vi "Epoch Library -- VI Tree.vi"() -> ()   [LabVIEW 2018]
uses:
  <vilib>/LabVIEW Open Source Project/Epoch Date & Time/Epochs -- enum.ctl
  <vilib>/LabVIEW Open Source Project/Epoch Date & Time/formatter.iso8601/ISO8601 Date Formats.ctl
  <vilib>/LabVIEW Open Source Project/Epoch Date & Time/Timestamp Compare Units -- enum.ctl
  <vilib>/LabVIEW Open Source Project/Epoch Date & Time/formatter.iso8601/DateTime.ISO8601.lvclass
  C:/Program Files (x86)/National Instruments/LabVIEW 2018/vi.lib/LabVIEW Open Source Project/Epoch Date & Time/formatter/DateTimeFormatter.lvclass
  <vilib>/LabVIEW Open Source Project/Epoch Date & Time/formatter.rfc5322/DateTime.RFC5322.lvclass
  <vilib>/LabVIEW Open Source Project/Epoch Date & Time/epoch/Epoch.lvclass
  <vilib>/LabVIEW Open Source Project/Epoch Date & Time/epoch.UTC/Epoch.UTC.lvclass
  <vilib>/LabVIEW Open Source Project/Epoch Date & Time/epoch.GPS/Epoch.GPS.lvclass
  C:/Program Files (x86)/National Instruments/LabVIEW 2018/vi.lib/LabVIEW Open Source Project/Epoch Date & Time/epoch/Epoch.lvclass
  <vilib>/LabVIEW Open Source Project/Epoch Date & Time/epoch.UNIX/Epoch.UNIX.lvclass
  <vilib>/LabVIEW Open Source Project/Epoch Date & Time/formatter.iso8601/DateTime.ISO8601.lvclass/DateTime.ISO8601.ctl
  <vilib>/LabVIEW Open Source Project/Epoch Date & Time/isLeapYear (timestamp).vi
  <vilib>/LabVIEW Open Source Project/Epoch Date & Time/isLeapYear (integer).vi
  <vilib>/LabVIEW Open Source Project/Epoch Date & Time/formatter/DateTimeFormatter.lvclass
panel:
  out "Valid RFC5332 Internet Date":bool
  out "UNIX Conversion":bool
  out "UNIX Time (s)":i64
  out "GPS Time (s)":i64
  out "GPS Conversion":bool
  out "RFC5322 Email DateTime String":string
  out "Timestamp":timestamp
  out "ISO Strings":string[](array[string])
  out "timestamps":timestamp[](array[timestamp]) format="%<%.3X %x>T"
  out "Fractional Seconds":dbl[](array[numeric])
  out "Epoch Times (s)":i64[](array[numeric])
  out "Epochs":T1[](array[typedef])=[enum."Local", enum."UTC", enum."Unix", enum."GPS"]
  out "is 2021 a Leap Year?":bool
  out "ISO Week-Day Notation":bool
  out "ISO DateTime Notation":bool
  out "ISO8601 UTC DateTime String":string
  out "Valid RFC3339 Dates":bool
  out "Valid ISO Dates":bool
  out "is 2020 a Leap Year?":bool
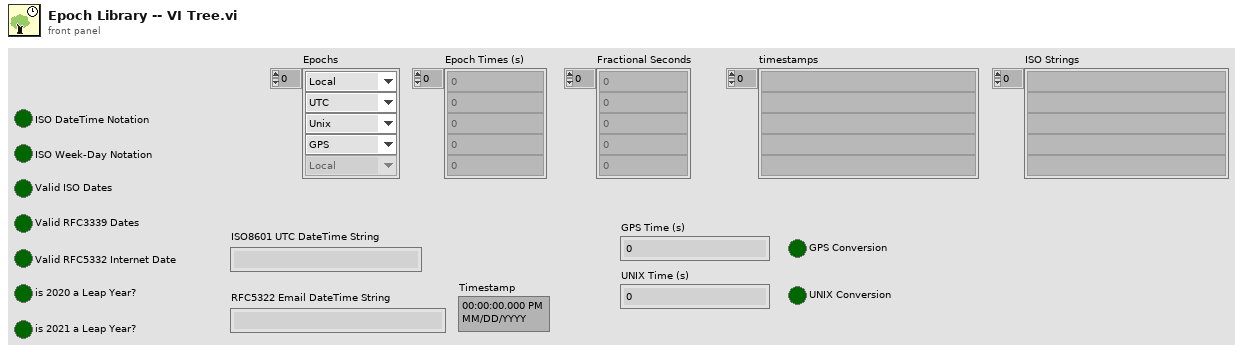
[diagram p1: front panel]
types:
  T1 = typedef "Epochs -- enum.ctl" = enum16{"Local", "UTC", "Unix", "GPS"}
  T2 = typedef "ISO8601 Date Formats.ctl" = enum16{"UTC Date-Time", "Date", "Calendar Month", "Week", "Week-Day", "Month-Day", "Ordinal Date"}
  T3 = typedef "Timestamp Compare Units -- enum.ctl" = enum16{"week", "day", "hour", "minute", "second", "millisecond", "microsecond", "nanosecond"}
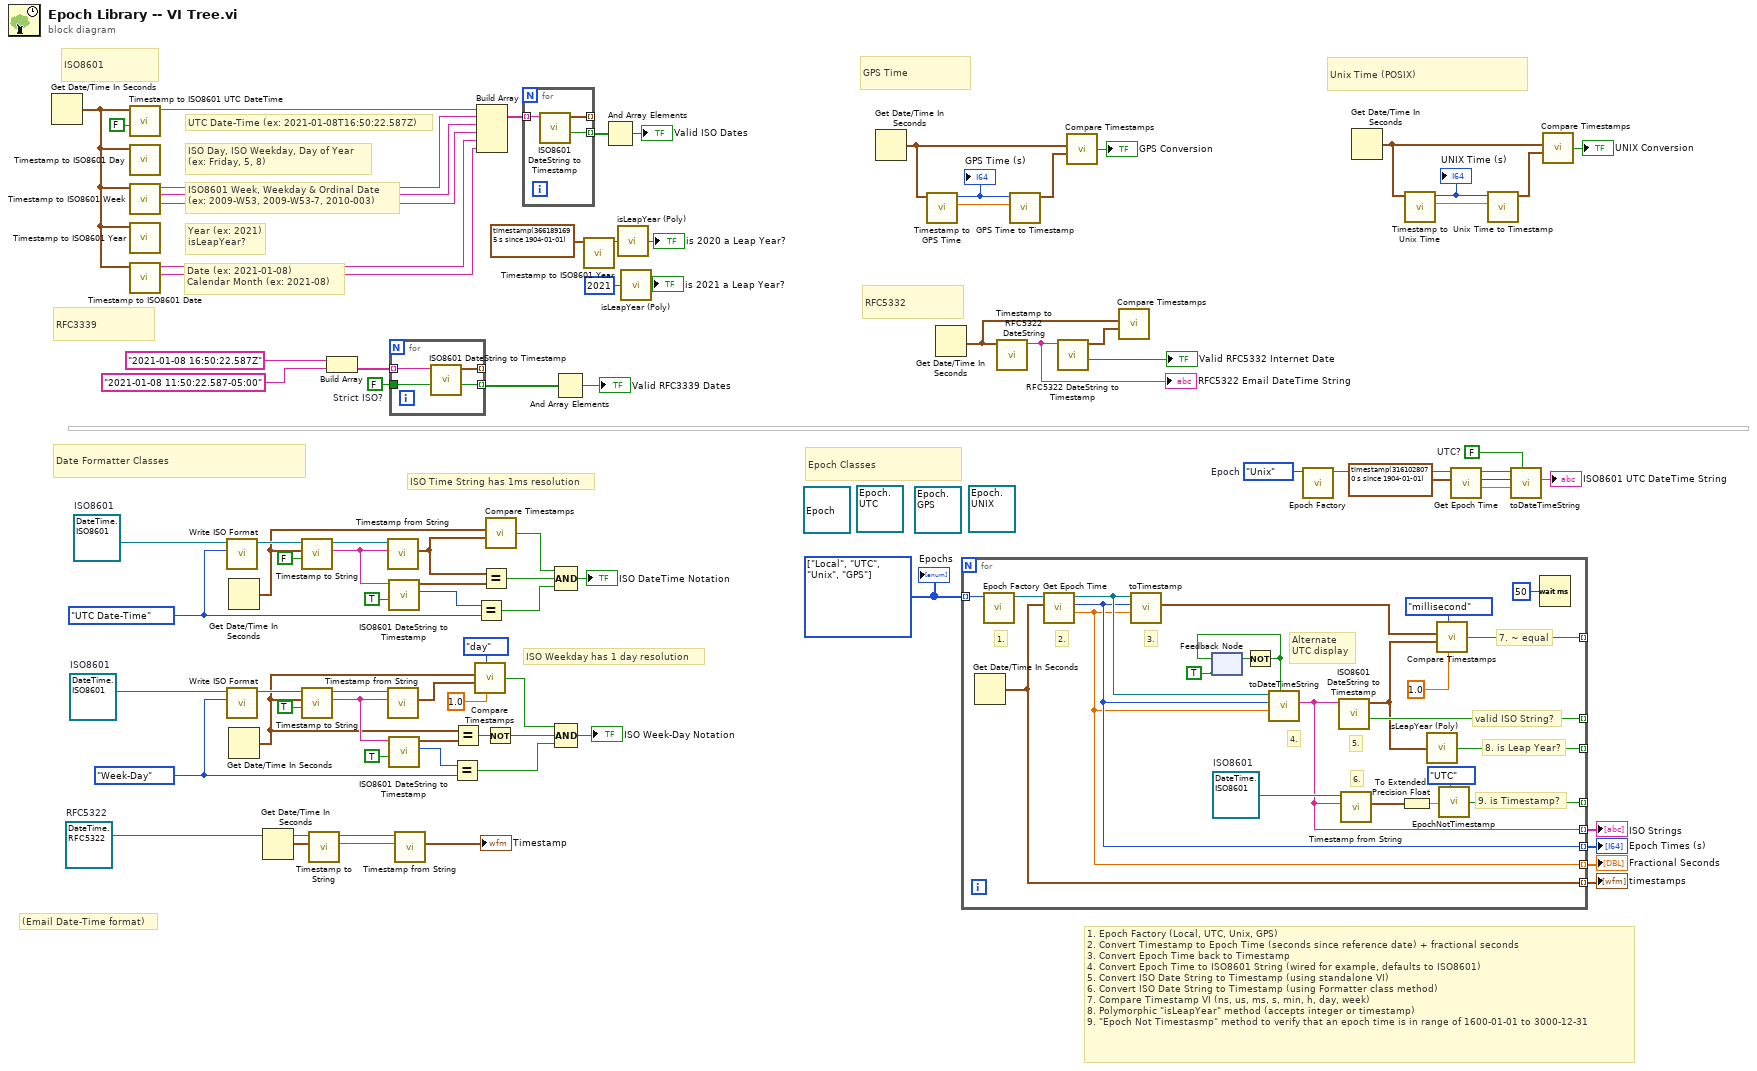
[diagram p0: block diagram]
diagram:
  (unwired) refnum<class "Epoch.UNIX.lvclass"> refnum ("Epoch.UNIX.lvclass")
  (unwired) refnum<class "Epoch.GPS.lvclass"> refnum ("Epoch.GPS.lvclass")
  (unwired) refnum<class "Epoch.UTC.lvclass"> refnum ("Epoch.UTC.lvclass")
  (unwired) refnum<class "Epoch.lvclass"> refnum ("Epoch.lvclass")
  w5 = T1[] [enum."Local", enum."UTC", enum."Unix", enum."GPS"] items=["Local", "UTC", "Unix", "GPS"]
  w6 = FALSE  # UTC?
  w13 = Epochs_--_enum."Unix"  # Epoch
  w43 = FALSE  # Strict ISO?
  w53 = refnum<class "DateTime.RFC5322.lvclass"> refnum  # RFC5322
  w73 = ISO8601_Date_Formats."Week-Day" ("ISO Format")
  w70 = refnum<class "DateTime.ISO8601.lvclass"> refnum  # ISO8601
  w80 = ISO8601_Date_Formats."UTC Date-Time" ("ISO Format")
  w83 = refnum<class "DateTime.ISO8601.lvclass"> refnum  # ISO8601
  # "Epoch Classes"
  # "1. Epoch Factory (Local, UTC, Unix, GPS)\n2. Convert Timestamp to Epoch Time (seconds since reference date) + fractional seconds\n3. Convert Epoch Time back to Timestamp\n4. Convert Epoch Time to ISO8601 String (wired for example, defaults to ISO8601)\n5. Convert ISO Date String to Timestamp (using standalone VI)\n6. Convert ISO Date String to Timestamp (using Formatter class method)\n7. Compare Timestamp VI (ns, us, ms, s, min, h, day, week)\n8. Polymorphic \"isLeapYear\" method (accepts integer or timestamp)\n9. \"Epoch Not Timestasmp\" method to verify that an epoch time is in range of 1600-01-01 to 3000-12-31"
  # "Date Formatter Classes"
  # "Unix Time (POSIX)"
  # "GPS Time"
  # "ISO8601"
  # "Date (ex: 2021-01-08)\nCalendar Month (ex: 2021-08)"
  # "Year (ex: 2021)\nisLeapYear?"
  # "ISO8601 Week, Weekday & Ordinal Date\n(ex: 2009-W53, 2009-W53-7, 2010-003)"
  # "ISO Day, ISO Weekday, Day of Year\n(ex: Friday, 5, 8)"
  # "UTC Date-Time (ex: 2021-01-08T16:50:22.587Z)"
  # "RFC3339"
  # "RFC5332"
  # "(Email Date-Time format)"
  # "ISO Weekday has 1 day resolution"
  # "ISO Time String has 1ms resolution"
  n1 = Get Date/Time In Seconds() -> (seconds since 1Jan1904=w38:timestamp)
  n2 = call <vilib>:"Timestamp to ISO8601 UTC DateTime.vi"("UTC? (F)"=FALSE, "Timestamp (now)"=w38) -> ("ISO8601 UTC DateTime"=w37:string)  [unwired: 9 in]
  n3 = call <vilib>:"Timestamp to ISO8601 Day.vi"("Timestamp (now)"=w38) -> ()  [unwired: 8 in, 3 out]
  n4 = call <vilib>:"Timestamp to ISO8601 Week.vi"("Timestamp (now)"=w38) -> ("ISO8601 Ordinal Date"=w34:string, "ISO8601 Weekday"=w35:string, "ISO8601 Week"=w36:string)  [unwired: 8 in]
  n5 = call <vilib>:"Timestamp to ISO8601 Year.vi"("Timestamp (now)"=w38) -> ()  [unwired: 9 in, 2 out]
  n6 = call <vilib>:"Timestamp to ISO8601 Date.vi"("Timestamp (now)"=w38) -> ("ISO8601 Calendar Month"=w32:string, "ISO8601 Date"=w33:string)  [unwired: 9 in]
  n7 = call <vilib>:"Write ISO Format.vi"("ISO Format"=w80, "DateTime.ISO8601 in"=w83) -> ("DateTime.ISO8601 out"=w84:refnum<class "DateTime.ISO8601.lvclass">)  [unwired: 9 in]
  n8 = call <vilib>:"Write ISO Format.vi"("ISO Format"=w73, "DateTime.ISO8601 in"=w70) -> ("DateTime.ISO8601 out"=w69:refnum<class "DateTime.ISO8601.lvclass">)  [unwired: 9 in]
  n9 = Get Date/Time In Seconds() -> (seconds since 1Jan1904=w55:timestamp)
  n10 = Get Date/Time In Seconds() -> (seconds since 1Jan1904=w65:timestamp)
  n11 = Get Date/Time In Seconds() -> (seconds since 1Jan1904=w51:timestamp)
  n12 = call <vilib>:"Timestamp to String.vi"("UTC? (F)"=FALSE, "Timestamp (now)"=w55, "DateTimeFormatter in"=w84) -> ("DateTime String"=w86:string, "DateTimeFormatter out"=w85:refnum<class "DateTime.ISO8601.lvclass">)  [unwired: 6 in, 1 out]
  n13 = call <vilib>:"Timestamp to String.vi"("UTC? (F)"=TRUE, "Timestamp (now)"=w65, "DateTimeFormatter in"=w69) -> ("DateTime String"=w67:string, "DateTimeFormatter out"=w68:refnum<class "DateTime.ISO8601.lvclass">)  [unwired: 6 in, 1 out]
  n14 = call <vilib>:"Timestamp to String.vi"("Timestamp (now)"=w51, "DateTimeFormatter in"=w53) -> ("DateTime String"=w52:string, "DateTimeFormatter out"=w54:refnum<class "DateTime.RFC5322.lvclass">)  [unwired: 7 in, 1 out]
  n15 = Build Array("2021-01-08 16:50:22.587Z" ("x"), "2021-01-08 11:50:22.587-05:00" ("x")) -> (w46:string[])
  n16 = call <vilib>:"Timestamp from String.vi"("DateTime String"=w86, "DateTimeFormatter in"=w85) -> ("Timestamp"=w56:timestamp)  [unwired: 7 in, 2 out]
  n17 = call <vilib>:"Timestamp from String.vi"("DateTime String"=w67, "DateTimeFormatter in"=w68) -> ("Timestamp"=w64:timestamp)  [unwired: 7 in, 2 out]
  n18 = call <vilib>:"ISO8601 DateString to Timestamp.vi"("Strict ISO? (T)"=TRUE, "ISO8601 Date String"=w86) -> ("ISO Format"=w81:T2, "Timestamp"=w82:timestamp)  [unwired: 7 in, 1 out]
  n19 = call <vilib>:"ISO8601 DateString to Timestamp.vi"("Strict ISO? (T)"=TRUE, "ISO8601 Date String"=w67) -> ("ISO Format"=w72:T2, "Timestamp"=w71:timestamp)  [unwired: 7 in, 1 out]
  n20 = for {
    tunnel: w46 -> [w91] mode=indexing
    tunnel: [w90] -> w45 mode=indexing
    tunnel: w43 -> [w89]
    tunnel: [w88] -> _ mode=indexing
    n21 = call <vilib>:"ISO8601 DateString to Timestamp.vi"("Strict ISO? (T)"=w89, "ISO8601 Date String"=w91) -> ("valid?"=w90:bool, "Timestamp"=w88:timestamp)  [unwired: 7 in, 1 out]
  }
  n22 = call <vilib>:"Timestamp from String.vi"("DateTime String"=w52, "DateTimeFormatter in"=w54) -> ("Timestamp"=→"Timestamp":timestamp)  [unwired: 7 in, 2 out]
  n23 = Equal?(x=w72, y=w73) -> (x = y?=w75:bool)
  n24 = Equal?(x=w65, y=w71) -> (x = y?=w74:bool)
  n25 = call <vilib>:"Compare Timestamps.vi"("Unit (ms)"=Timestamp_Compare_Units_--_enum."day" ("Unit (second)"), "timestamp (1)"=w65, "timestamp (2)"=w64, "Resolution (in selected unit)"=1.0) -> ("Equal?"=w63:bool)  [unwired: 4 in]
  n26 = Equal?(x=w81, y=w80) -> (x = y?=w78:bool)
  n27 = Build Array(w37, w36, w35, w34, w33, w32) -> (w31:string[])
  n28 = Equal?(x=w56, y=w82) -> (x = y?=w79:bool)
  n29 = Not(x=w74) -> (.not. x?=w62:bool)
  n30 = call <vilib>:"Compare Timestamps.vi"("timestamp (1)"=w55, "timestamp (2)"=w56) -> ("Equal?"=w57:bool)  [unwired: 6 in]
  n31 = for {
    tunnel: w31 -> [w94] mode=indexing
    tunnel: [w93] -> w30 mode=indexing
    tunnel: [w92] -> _ mode=indexing
    n32 = call <vilib>:"ISO8601 DateString to Timestamp.vi"("ISO8601 Date String"=w94) -> ("valid?"=w93:bool, "Timestamp"=w92:timestamp)  [unwired: 8 in, 1 out]
  }
  n33 = And Array Elements(Boolean array=w45) -> (logical AND=→"Valid RFC3339 Dates":bool)
  n34 = Compound Arithmetic op=AND(w57, w79, w78) -> (→"ISO DateTime Notation":bool)
  n35 = Compound Arithmetic op=AND(w63, w62, w75) -> (→"ISO Week-Day Notation":bool)
  n36 = call <vilib>:"Timestamp to ISO8601 Year.vi"("Timestamp (now)"=timestamp(3661891695.389395 s since 1904-01-01)) -> ("year"=w29:i32)  [unwired: 9 in, 1 out]
  n37 = And Array Elements(Boolean array=w30) -> (logical AND=→"Valid ISO Dates":bool)
  n38 = call-poly <vilib>:"isLeapYear (Poly).vi"("Year (0: this year)"=w29) -> ("is Leap Year?"=→"is 2020 a Leap Year?":bool)  [unwired: 8 in]
  n39 = call-poly <vilib>:"isLeapYear (Poly).vi"("Year (0: this year)"=2021) -> ("is Leap Year?"=→"is 2021 a Leap Year?":bool)  [unwired: 8 in]
  n40 = Get Date/Time In Seconds() -> (seconds since 1Jan1904=w22:timestamp)
  n41 = call <vilib>:"Timestamp to GPS Time.vi"("Timestamp (now)"=w22) -> ("Fractional Second"=w20:dbl, "GPS Time (s)"=w19:i64)  [unwired: 9 in]
  "GPS Time (s)" <- w19
  n42 = Get Date/Time In Seconds() -> (seconds since 1Jan1904=w47:timestamp)
  n43 = for {
    tunnel: w5 -> [w117] mode=indexing
    tunnel: [w113] -> _ mode=indexing
    tunnel: [w110] -> _ mode=indexing
    tunnel: [w109] -> _ mode=indexing
    tunnel: [w106] -> _ mode=indexing
    tunnel: [w105] -> w4 mode=indexing
    tunnel: [w104] -> w3 mode=indexing
    tunnel: [w98] -> w2 mode=indexing
    tunnel: [w102] -> w1 mode=indexing
    w111 = refnum<class "DateTime.ISO8601.lvclass"> refnum  # ISO8601
    # "Alternate\nUTC display"
    # "6."
    # "5."
    # "9. is Timestamp?"
    # "8. is Leap Year?"
    # "valid ISO String?"
    # "7. ~ equal"
    # "4."
    # "3."
    # "2."
    # "1."
    n44 = Get Date/Time In Seconds() -> (seconds since 1Jan1904=w98:timestamp)
    n45 = call <vilib>:"Epoch Factory.vi"("Epoch (Local System)"=w117) -> ("Epoch object"=w116:refnum<class "Epoch.lvclass">)  [unwired: 10 in]
    n46 = call <vilib>:"Get Epoch Time.vi"("Timestamp (now)"=w98, "Epoch (Local)"=w116) -> ("Fractional Second"=w104:dbl, "Epoch Time (s)"=w105:i64, "Epoch out"=w112:refnum<class "Epoch.lvclass">)  [unwired: 7 in]
    n47 = call-dynamic "toTimestamp.vi"("Fractional Second"=w104, "Epoch Time (s)"=w105, "Epoch (Local)"=w112) -> ("Timestamp"=w97:timestamp)  [unwired: 6 in, 2 out]
    n48 = feedback #1(TRUE) -> (w100:bool)
    n49 = Not(x=w100) -> (.not. x?=w99:bool)
    n50 = feedback-in #1(w99) -> ()
    n51 = call <vilib>:"toDateTimeString.vi"("UTC? (F)"=w99, "Fractional Second"=w104, "Epoch Time (s)"=w105, "Epoch"=w112) -> ("DateTime string"=w102:string)  [unwired: 5 in, 2 out]
    n52 = call <vilib>:"ISO8601 DateString to Timestamp.vi"("ISO8601 Date String"=w102) -> ("valid?"=w110:bool, "Timestamp"=w96:timestamp)  [unwired: 8 in, 1 out]
    n53 = call <vilib>:"Timestamp from String.vi"("DateTime String"=w102, "DateTimeFormatter in"=w111) -> ("Timestamp"=w95:timestamp)  [unwired: 7 in, 2 out]
    n54 = To Extended Precision Float(1:w95) -> (0:w108:ext)
    n55 = call-poly <vilib>:"isLeapYear (Poly).vi"("timestamp (now)"=w96) -> ("is Leap Year?"=w109:bool)  [unwired: 8 in]
    n56 = call <vilib>:"Compare Timestamps.vi"("Unit (ms)"=Timestamp_Compare_Units_--_enum."millisecond" ("Unit (second)"), "timestamp (1)"=w97, "timestamp (2)"=w96, "Resolution (in selected unit)"=1.0) -> ("Equal?"=w113:bool)  [unwired: 4 in]
    n57 = call <vilib>:"EpochNotTimestamp.vi"("Epoch (UTC)"=Epochs_--_enum."UTC", "Epoch Time"=w108) -> ("Not a Timestamp?"=w106:bool)  [unwired: 7 in]
    n58 = Wait (ms)(milliseconds to wait=u32 50) -> ()  [unwired: 1 out]
  }
  "Epoch Times (s)" <- w4
  "Fractional Seconds" <- w3
  "timestamps" <- w2
  "ISO Strings" <- w1
  n59 = call <vilib>:"Timestamp to RFC5322 DateString.vi"("Timestamp (now)"=w47) -> ("RFC5322 Date String"=w49:string)  [unwired: 10 in]
  "RFC5322 Email DateTime String" <- w49
  n60 = call <vilib>:"GPS Time to Timestamp.vi"("Fractional Second"=w20, "GPS Time (s)"=w19) -> ("Timestamp"=w21:timestamp)  [unwired: 8 in, 1 out]
  n61 = call <vilib>:"RFC5322 DateString to Timestamp.vi"("RFC5322 Date String"=w49) -> ("valid?"=→"Valid RFC5332 Internet Date":bool, "Timestamp"=w48:timestamp)  [unwired: 8 in, 1 out]
  n62 = call <vilib>:"Compare Timestamps.vi"("timestamp (1)"=w22, "timestamp (2)"=w21) -> ("Equal?"=→"GPS Conversion":bool)  [unwired: 6 in]
  n63 = call <vilib>:"Compare Timestamps.vi"("timestamp (1)"=w47, "timestamp (2)"=w48) -> ()  [unwired: 6 in, 1 out]
  n64 = call <vilib>:"Epoch Factory.vi"("Epoch (Local System)"=w13) -> ("Epoch object"=w12:refnum<class "Epoch.lvclass">)  [unwired: 10 in]
  n65 = Get Date/Time In Seconds() -> (seconds since 1Jan1904=w17:timestamp)
  n66 = call <vilib>:"Timestamp to Unix Time.vi"("Timestamp (now)"=w17) -> ("Fractional Second"=w15:dbl, "Unix Time (s)"=w16:i64)  [unwired: 9 in]
  "UNIX Time (s)" <- w16
  n67 = call <vilib>:"Get Epoch Time.vi"("Timestamp (now)"=timestamp(3161028070.7687225 s since 1904-01-01), "Epoch (Local)"=w12) -> ("Fractional Second"=w11:dbl, "Epoch Time (s)"=w10:i64, "Epoch out"=w9:refnum<class "Epoch.lvclass">)  [unwired: 7 in]
  n68 = call <vilib>:"Unix Time to Timestamp.vi"("Fractional Second"=w15, "Unix Time (s)"=w16) -> ("Timestamp"=w14:timestamp)  [unwired: 8 in, 1 out]
  n69 = call <vilib>:"toDateTimeString.vi"("UTC? (F)"=w6, "Fractional Second"=w11, "Epoch Time (s)"=w10, "Epoch"=w9) -> ("DateTime string"=→"ISO8601 UTC DateTime String":string)  [unwired: 5 in, 2 out]
  n70 = call <vilib>:"Compare Timestamps.vi"("timestamp (1)"=w17, "timestamp (2)"=w14) -> ("Equal?"=→"UNIX Conversion":bool)  [unwired: 6 in]
  "Epochs" <- w5
